vi "Lab_JouleScope.vi"() -> ()   [LabVIEW 2015]
uses:
  Ctrl/I_range.ctl
  Ctrl/R_W.ctl
  <vilib>/Analysis/3filter.llb/Filter Passband Type.ctl
  SubVIs/JSON_send/Send_JSN_Message_2 (SubVI).vi
  SubVIs/JSON_send/Send_JSN_Message_0 (SubVI).vi
  SubVIs/JSON_extract_data/JSON_extract_Data_2 (SubVI).vi
  SubVIs/JSON_extract_data/JSON_extract_Data_1 (SubVI).vi
  SubVIs/JSON_send/Send_JSN_Message_1 (SubVI).vi
  SubVIs/JSON_extract_data/JSON_extract_Data_7 (SubVI).vi
  SubVIs/JSON_extract_data/JSON_extract_Data_6 (SubVI).vi
  SubVIs/JSON_send/Send_JSN_Message_7 (SubVI).vi
  SubVIs/JSON_extract_data/JSON_extract_Data_4 (SubVI).vi
  <vilib>/Analysis/3filter.llb/Butterworth Filter (DBL).vi
  <vilib>/Analysis/NI_AALBase.lvlib
panel:
  out "Stop_Var":bool=TRUE
  in  "Tab Control":enum32{"Init", "Visu"}(tab)=enum."Visu"
  out "Device":string="Joulescope:001747"
  out "Parameters":string="{\"type\": \"parameters\", \"phase\": \"rsp\", \"id\": 3, \"status\": 200, \"status_msg\": \"Success\", \"device\": \"Joulescope:001747\", \"data\": {\"sensor_power\": {\"name\": \"sensor_power\", \"default\": \"on\", \"path\": \"setting\", \"options\": [[\"off\", 0, []], [\"on\", 1, []]], \"units\": null, \"brief\": \"Force the sensor power on or off.\", \"detail\": \"Altering this parameter during operation may cause errors.\", \"flags\": [\"developer\"]}, \"source\": {\"name\": \"source\", \"default\": \"off\", \"path\": \"setting\", \"options\": [[\"off\", 0, []], [\"raw\", 192, [\"on\"]], [\"pattern_usb\", 9, []], [\"pattern_control\", 10, []], [\"pattern_sensor\", 175, []]], \"units\": null, \"brief\": \"Select the streaming data source.\", \"detail\": null, \"flags\": [\"developer\"]}, \"i_range\": {\"name\": \"i_range\", \"default\": \"off\", \"path\": \"setting\", \"options\": [[\"auto\", 128, [\"on\"]], [\"10 A\", 1, [\"0\", 0]], [\"2 A\", 2, [\"1\", 1]], [\"180 mA\", 4, [\"2\", 2]], [\"18 mA\", 8, [\"3\", 3]], [\"1.8 mA\", 16, [\"4\", 4]], [\"180 \\u00b5A\", 32, [\"5\", 5]], [\"18 \\u00b5A\", 64, [\"6\", 6]], [\"off\", 0, []]], \"units\": null, \"brief\": \"Select the current measurement range (shunt resistor)\", \"detail\": null, \"flags\": []}, \"v_range\": {\"name\": \"v_range\", \"default\": \"15V\", \"path\": \"setting\", \"options\": [[\"15V\", 0, [\"low\", 0]], [\"5V\", 1, [\"high\", 1]]], \"units\": null, \"brief\": \"Select the voltage measurement range (gain)\", \"detail\": null, \"flags\": []}, \"ovr_to_lsb\": {\"name\": \"ovr_to_lsb\", \"default\": \"off\", \"path\": \"setting\", \"options\": [[\"off\", 0, []], [\"on\", 1, []]], \"units\": null, \"brief\": \"Map overflow flags to the LSBs\", \"detail\": null, \"flags\": [\"developer\"]}, \"trigger_source\": {\"name\": \"trigger_source\", \"default\": \"auto\", \"path\": \"extio\", \"options\": [[\"auto\", 0, []], [\"gpi0\", 2, []], [\"gpi1\", 3, []]], \"units\": null, \"brief\": \"Select the trigger source\", \"detail\": null, \"flags\": [\"hidden\"]}, \"io_voltage\": {\"name\": \"io_voltage\", \"default\": \"3.3V\", \"path\": \"extio\", \"options\": [[\"1.8V\", 1800, []], [\"2.1V\", 2100, []], [\"2.5V\", 2500, []], [\"2.7V\", 2700, []], [\"3.0V\", 3000, []], [\"3.3V\", 3300, []], [\"3.6V\", 3600, []], [\"5.0V\", 5000, []]], \"units\": null, \"brief\": \"The GPI/O high-level voltage.\", \"detail\": null, \"flags\": []}, \"gpo0\": {\"name\": \"gpo0\", \"default\": \"0\", \"path\": \"extio\", \"options\": [[\"0\", 0, [0]], [\"1\", 1, [1]]], \"units\": null, \"brief\": \"The GPO bit 0 output value.\", \"detail\": null, \"flags\": []}, \"gpo1\": {\"name\": \"gpo1\", \"default\": \"0\", \"path\": \"extio\", \"options\": [[\"0\", 0, [0]], [\"1\", 1, [1]]], \"units\": null, \"brief\": \"The GPO bit 1 output value.\", \"detail\": null, \"flags\": []}, \"current_lsb\": {\"name\": \"current_lsb\", \"default\": \"normal\", \"path\": \"extio\", \"options\": [[\"normal\", 0, []], [\"gpi0\", 2, []], [\"gpi1\", 3, []]], \"units\": null, \"brief\": \"The current signal least-significant bit mapping.\", \"detail\": null, \"flags\": []}, \"voltage_lsb\": {\"name\": \"voltage_lsb\", \"default\": \"normal\", \"path\": \"extio\", \"options\": [[\"normal\", 0, []], [\"gpi0\", 2, []], [\"gpi1\", 3, []]], \"units\": null, \"brief\": \"The voltage signal least-significant bit mapping.\", \"detail\": null, \"flags\": []}, \"control_test_mode\": {\"name\": \"control_test_mode\", \"default\": \"normal\", \"path\": \"setting\", \"options\": [[\"normal\", 3, []], [\"usb\", 129, []], [\"fpga\", 130, []], [\"both\", 131, []]], \"units\": null, \"brief\": \"Set the test mode\", \"detail\": null, \"flags\": [\"developer\"]}, \"transfer_length\": {\"name\": \"transfer_length\", \"default\": \"256\", \"path\": \"setting\", \"options\": [[\"1\", 1, []], [\"2\", 2, []], [\"4\", 4, []], [\"8\", 8, []], [\"16\", 16, []], [\"32\", 32, []], [\"64\", 64, []], [\"128\", 128, []], [\"256\", 256, []]], \"units\": \"packets\", \"brief\": \"Set the USB transfer length in packets\", \"detail\": null, \"flags\": [\"developer\", \"skip_update\"]}, \"transfer_outstanding\": {\"name\": \"transfer_outstanding\", \"default\": \"8\", \"path\": \"setting\", \"options\": [[\"1\", 1, []], [\"2\", 2, []], [\"4\", 4, []], [\"8\", 8, []]], \"units\": null, \"brief\": \"Set the maximum number of USB transfers issued simultaneously\", \"detail\": null, \"flags\": [\"developer\", \"skip_update\"]}, \"current_ranging\": {\"name\": \"current_ranging\", \"default\": null, \"path\": \"current_ranging\", \"options\": [], \"units\": null, \"brief\": null, \"detail\": null, \"flags\": [\"hidden\"]}, \"current_ranging_type\": {\"name\": \"current_ranging_type\", \"default\": \"interp\", \"path\": \"current_ranging\", \"options\": [[\"off\", \"off\", []], [\"mean\", \"mean\", []], [\"interp\", \"interp\", [\"interpolate\"]], [\"NaN\", \"nan\", [\"nan\"]]], \"units\": null, \"brief\": \"The filter type.\", \"detail\": null, \"flags\": []}, \"current_ranging_samples_pre\": {\"name\": \"current_ranging_samples_pre\", \"default\": \"1\", \"path\": \"current_ranging\", \"options\": [[\"0\", 0, [0]], [\"1\", 1, [1]], [\"2\", 2, [2]], [\"3\", 3, [3]], [\"4\", 4, [4]], [\"5\", 5, [5]], [\"6\", 6, [6]], [\"7\", 7, [7]], [\"8\", 8, [8]]], \"units\": null, \"brief\": \"The number of samples before the range switch to include.\", \"detail\": \"Only valid for type \\\"mean\\\" - ignored for \\\"off\\\", \\\"interp\\\", and \\\"NaN\\\".\", \"flags\": []}, \"current_ranging_samples_window\": {\"name\": \"current_ranging_samples_window\", \"default\": \"n\", \"path\": \"current_ranging\", \"options\": [[\"m\", \"m\", []], [\"n\", \"n\", []], [\"0\", 0, [0]], [\"1\", 1, [1]], [\"2\", 2, [2]], [\"3\", 3, [3]], [\"4\", 4, [4]], [\"5\", 5, [5]], [\"6\", 6, [6]], [\"7\", 7, [7]], [\"8\", 8, [8]], [\"9\", 9, [9]], [\"10\", 10, [10]], [\"11\", 11, [11]], [\"12\", 12, [12]]], \"units\": null, \"brief\": \"The number of samples to adjust.\", \"detail\": \"Use \\\"n\\\" for automatic duration based upon known response time. Use \\\"m\\\" for shorter automatic duration that may result in min/max distortion.\", \"flags\": []}, \"current_ranging_samples_post\": {\"name\": \"current_ranging_samples_post\", \"default\": \"1\", \"path\": \"current_ranging\", \"options\": [[\"0\", 0, [0]], [\"1\", 1, [1]], [\"2\", 2, [2]], [\"3\", 3, [3]], [\"4\", 4, [4]], [\"5\", 5, [5]], [\"6\", 6, [6]], [\"7\", 7, [7]], [\"8\", 8, [8]]], \"units\": null, \"brief\": \"The number of samples after the range switch to include.\", \"detail\": \"Only valid for type \\\"mean\\\" - ignored for \\\"off\\\", \\\"interp\\\", and \\\"NaN\\\".\", \"flags\": []}, \"buffer_duration\": {\"name\": \"buffer_duration\", \"default\": \"30 seconds\", \"path\": \"setting\", \"options\": [[\"15 seconds\", 15, [15]], [\"30 seconds\", 30, [30]], [\"1 minute\", 60, [60]], [\"2 minutes\", 120, [120]], [\"5 minutes\", 300, [300]], [\"10 minutes\", 600, [600]], [\"20 minutes\", 1200, [1200]], [\"1 hour\", 3600, [3600]], [\"2 hours\", 7200, [7200]], [\"5 hours\", 18000, [18000]], [\"10 hours\", 36000, [36000]], [\"1 day\", 86400, [86400]]], \"units\": \"seconds\", \"brief\": \"The amount of sample data to store in memory.\", \"detail\": \"Use care when setting this value. The software requires 1.5 GB of RAM for every 60 seconds at the full 2 MSPS rate.\", \"flags\": [\"skip_update\"]}, \"reduction_frequency\": {\"name\": \"reduction_frequency\", \"default\": \"2 Hz\", \"path\": \"setting\", \"options\": [[\"100 Hz\", 100, [100]], [\"50 Hz\", 50, [50]], [\"20 Hz\", 20, [20]], [\"10 Hz\", 10, [10]], [\"5 Hz\", 5, [5]], [\"2 Hz\", 2, [2]], [\"1 Hz\", 1, [1]]], \"units\": \"Hz\", \"brief\": \"The rate that the device produces statistics, including multimeter values.\", \"detail\": null, \"flags\": [\"skip_update\"]}, \"sampling_frequency\": {\"name\": \"sampling_frequency\", \"default\": \"2 MHz\", \"path\": \"setting\", \"options\": [[\"2 MHz\", 2000000, [2000000, \"auto\", null, \"default\"]], [\"1 MHz\", 1000000, [1000000]], [\"500 kHz\", 500000, [500000]], [\"200 kHz\", 200000, [200000]], [\"100 kHz\", 100000, [100000]], [\"50 kHz\", 50000, [50000]], [\"20 kHz\", 20000, [20000]], [\"10 kHz\", 10000, [10000]], [\"5 kHz\", 5000, [5000]], [\"2 kHz\", 2000, [2000]], [\"1 kHz\", 1000, [1000]], [\"500 Hz\", 500, [500]], [\"200 Hz\", 200, [200]], [\"100 Hz\", 100, [100]], [\"50 Hz\", 50, [50]], [\"20 Hz\", 20, [20]], [\"10 Hz\", 10, [10]]], \"units\": \"Hz\", \"brief\": \"The rate that the device produces samples.\", \"detail\": null, \"flags\": [\"skip_update\"]}, \"model\": {\"name\": \"model\", \"default\": null, \"path\": \"info\", \"options\": [], \"units\": null, \"brief\": null, \"detail\": null, \"flags\": [\"read_only\", \"hidden\"]}, \"device_serial_number\": {\"name\": \"device_serial_number\", \"default\": null, \"path\": \"info\", \"options\": [], \"units\": null, \"brief\": null, \"detail\": null, \"flags\": [\"read_only\", \"hidden\"]}, \"hardware_serial_number\": {\"name\": \"hardware_serial_number\", \"default\": null, \"path\": \"info\", \"options\": [], \"units\": null, \"brief\": null, \"detail\": null, \"flags\": [\"read_only\", \"hidden\"]}}}"
  out "Infos":T1={"protocol_version"=1, "server_version"="0.1.2", "joulescope_version"="0.9.7"}
  out "infos":string="{\"type\": \"info\", \"phase\": \"rsp\", \"id\": 4, \"status\": 200, \"status_msg\": \"Success\", \"device\": \"Joulescope:001747\", \"data\": {\"type\": \"info\", \"ver\": 1, \"ctl\": {\"mfg\": {\"country\": \"USA\", \"location\": \"MD_01\", \"lot\": \"202043_00\"}, \"hw\": {\"rev\": \"H\", \"sn_mcu\": \"510D00D070D4A1BA683523C52091005F\", \"sn_mfg\": \"001747\"}, \"fw\": {\"ver\": \"1.3.2\"}, \"fpga\": {\"ver\": \"0.2.0\", \"prod_id\": \"0x9314acf2\"}}, \"sensor\": {\"fw\": {\"ver\": \"1.3.2\"}, \"fpga\": {\"ver\": \"1.2.1\"}}}}"
  out "OK raw data":bool=TRUE
  in  "i_range request_1":cluster{"name":string, "value":T2}={"name"="i_range", "value"=enum."1.8 mA"}
  out "Current":sgl[](graph)
  out "Voltage":sgl[](graph)
  in  "fc":dbl=2000.0 format="%#_13g"
  in  "stop":bool
  out "i_range":string="1.8 mA"
  out "statistiques":string="{\"type\": \"statistics\", \"phase\": \"async\", \"device\": \"Joulescope:001747\", \"data\": {\"time\": {\"range\": {\"value\": [29.0, 29.5], \"units\": \"s\"}, \"delta\": {\"value\": 0.5, \"units\": \"s\"}, \"samples\": {\"value\": 1000000, \"units\": \"samples\"}, \"sample_range\": {\"value\": [58000000, 59000000], \"units\": \"input_samples\"}}, \"signals\": {\"current\": {\"\\u00b5\": {\"value\": 2.5195384097245923e-06, \"units\": \"A\"}, \"\\u03c32\": {\"value\": 1.3499273425982267e-11, \"units\": \"A\"}, \"min\": {\"value\": -1.4949010619602632e-05, \"units\": \"A\"}, \"max\": {\"value\": 3.776274752453901e-05, \"units\": \"A\"}, \"p2p\": {\"value\": 5.271175814414164e-05, \"units\": \"A\"}, \"\\u222b\": {\"value\": 1.2597692048622961e-06, \"units\": \"C\"}}, \"voltage\": {\"\\u00b5\": {\"value\": 2.988984020348548, \"units\": \"V\"}, \"\\u03c32\": {\"value\": 1.098181211591936e-06, \"units\": \"V\"}, \"min\": {\"value\": 2.984358787536621, \"units\": \"V\"}, \"max\": {\"value\": 2.993438720703125, \"units\": \"V\"}, \"p2p\": {\"value\": 0.009079933166503906, \"units\": \"V\"}}, \"power\": {\"\\u00b5\": {\"value\": 7.5309005292030786e-06, \"units\": \"W\"}, \"\\u03c32\": {\"value\": 1.206049847016679e-10, \"units\": \"W\"}, \"min\": {\"value\": -4.4664109736913815e-05, \"units\": \"W\"}, \"max\": {\"value\": 0.00011286902736173943, \"units\": \"W\"}, \"p2p\": {\"value\": 0.00015753313709865324, \"units\": \"W\"}, \"\\u222b\": {\"value\": 3.7654502646015393e-06, \"units\": \"J\"}}, \"current_range\": {\"\\u00b5\": {\"value\": 4.0, \"units\": \"\"}, \"\\u03c32\": {\"value\": 0.0, \"units\": \"\"}, \"min\": {\"value\": 4.0, \"units\": \"\"}, \"max\": {\"value\": 4.0, \"units\": \"\"}, \"p2p\": {\"value\": 0.0, \"units\": \"\"}}, \"current_lsb\": {\"\\u00b5\": {\"value\": 0.5333319999999999, \"units\": \"\"}, \"\\u03c32\": {\"value\": 0.24888922666522673, \"units\": \"\"}, \"min\": {\"value\": 0.0, \"units\": \"\"}, \"max\": {\"value\": 1.0, \"units\": \"\"}, \"p2p\": {\"value\": 1.0, \"units\": \"\"}}, \"voltage_lsb\": {\"\\u00b5\": {\"value\": 0.5333329999999997, \"units\": \"\"}, \"\\u03c32\": {\"value\": 0.24888916000015993, \"units\": \"\"}, \"min\": {\"value\": 0.0, \"units\": \"\"}, \"max\": {\"value\": 1.0, \"units\": \"\"}, \"p2p\": {\"value\": 1.0, \"units\": \"\"}}}, \"source\": \"stream_buffer\", \"accumulators\": {\"charge\": {\"value\": 7.7435459e-05, \"units\": \"C\"}, \"energy\": {\"value\": 0.00023147490999999998, \"units\": \"J\"}}}, \"status\": 200, \"status_msg\": \"Success\"}"
  # "Lab_JouleScope"
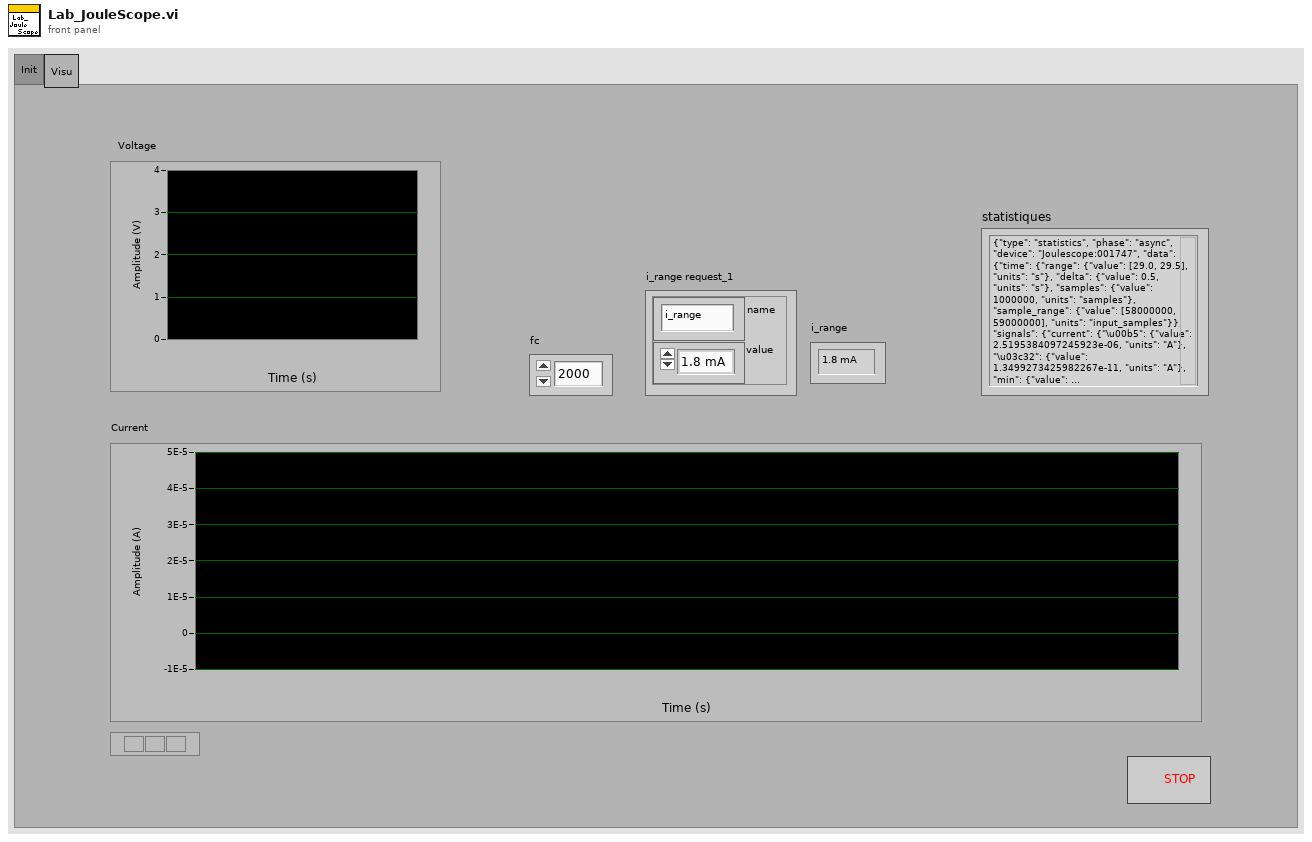
[diagram p1: front panel]
types:
  T1 = cluster{"protocol_version":i32, "server_version":string, "joulescope_version":string}
  T2 = typedef "I_range.ctl" = enum16{"off", "18 µA", "180 µA", "1.8 mA", "18 mA", "180 mA", "2 A", "10 A", "auto"}
  T3 = typedef "R_W.ctl" = enum16{"Write", "Read", "RAZ"}
  T4 = typedef "NI_AALBase.lvlib/Filter Passband Type.ctl" = enum32{"Lowpass", "Highpass", "Bandpass", "Bandstop"}
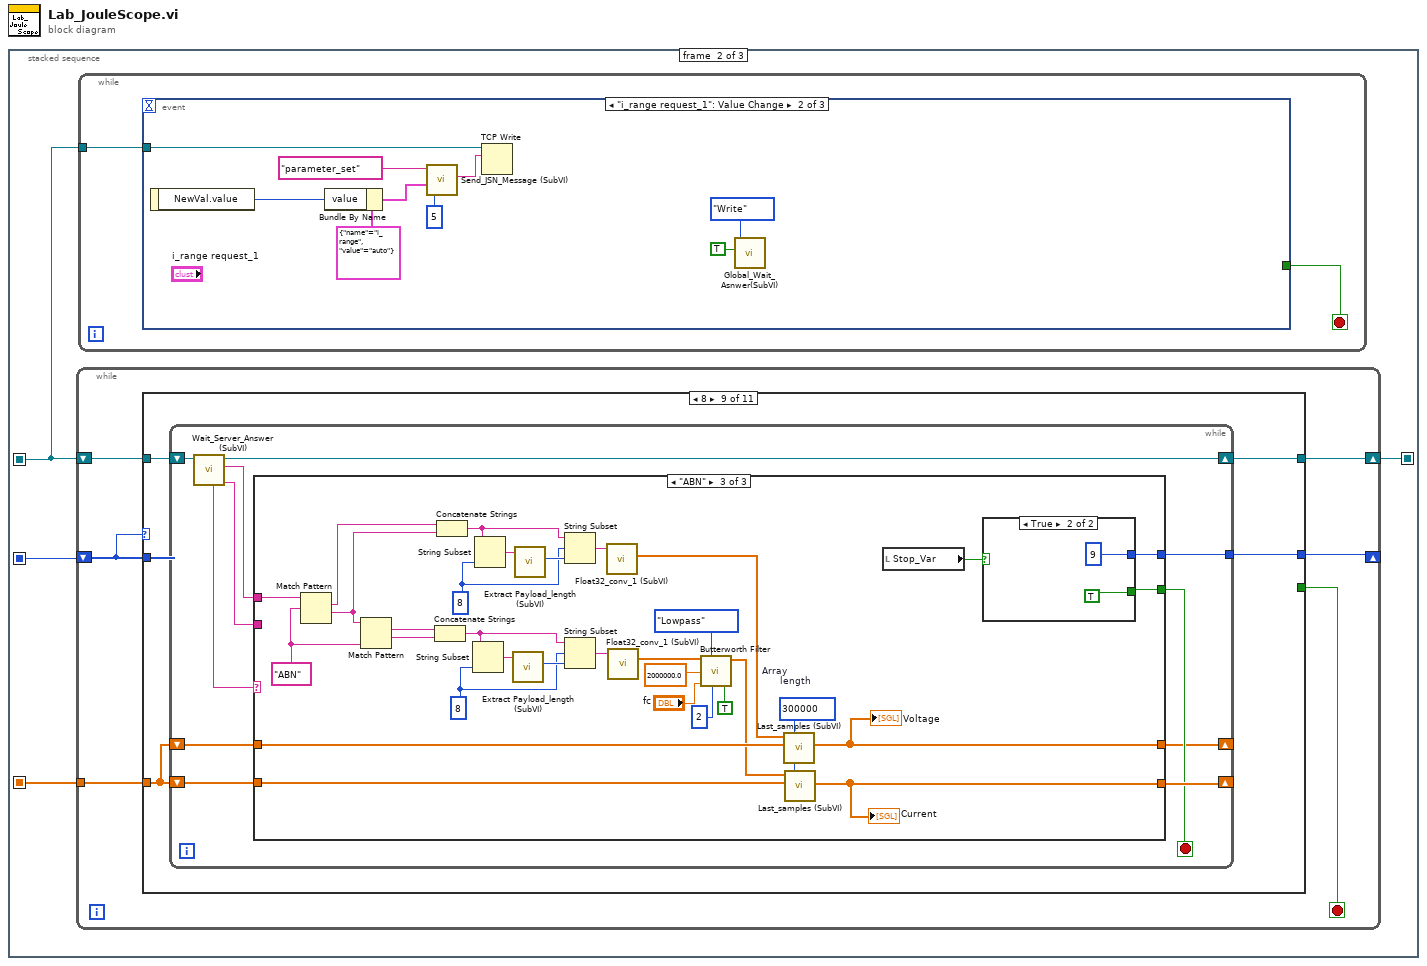
[diagram p0: block diagram]
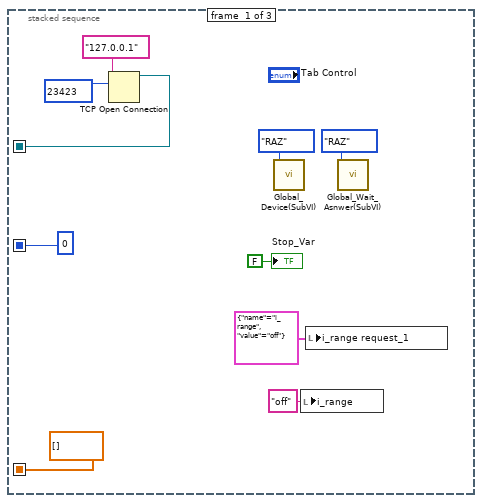
[diagram p2: hidden frame]
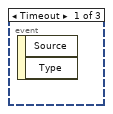
[diagram p3: hidden frame]
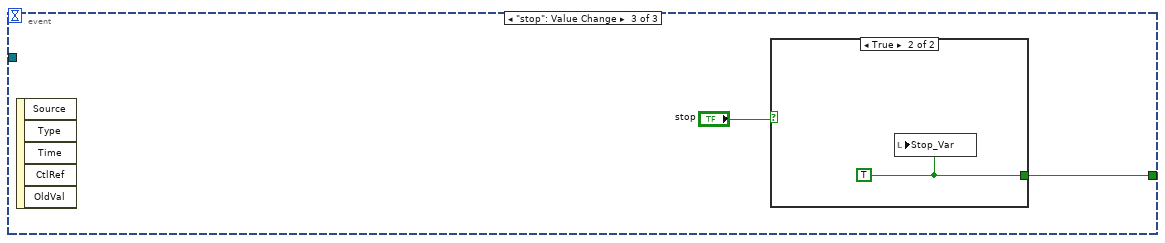
[diagram p4: hidden frame]
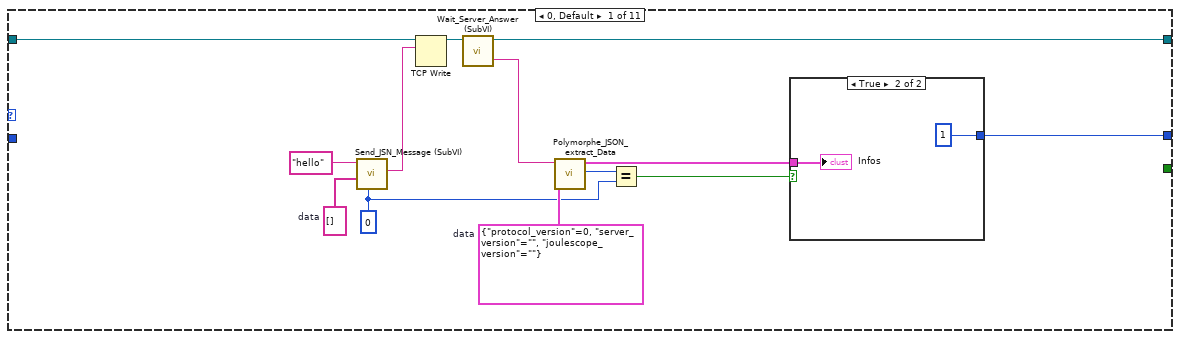
[diagram p6: hidden frame]
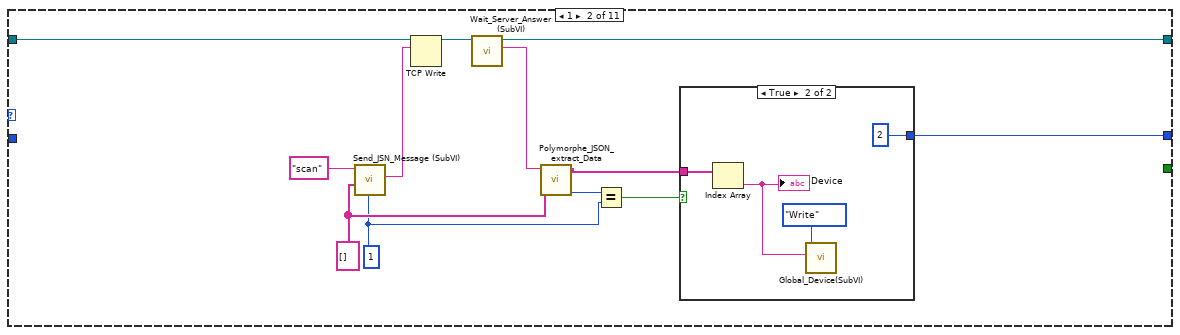
[diagram p8: hidden frame]
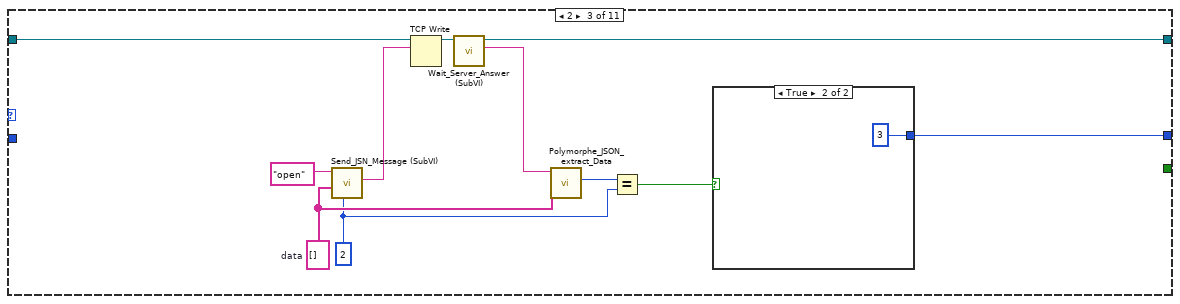
[diagram p10: hidden frame]
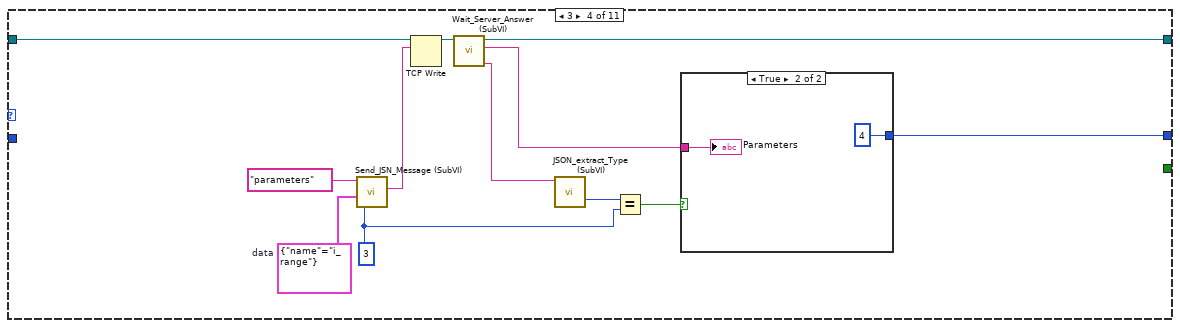
[diagram p12: hidden frame]
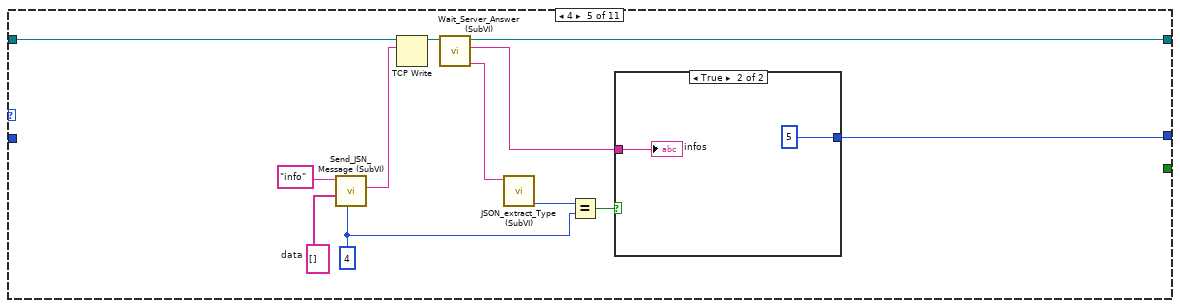
[diagram p14: hidden frame]
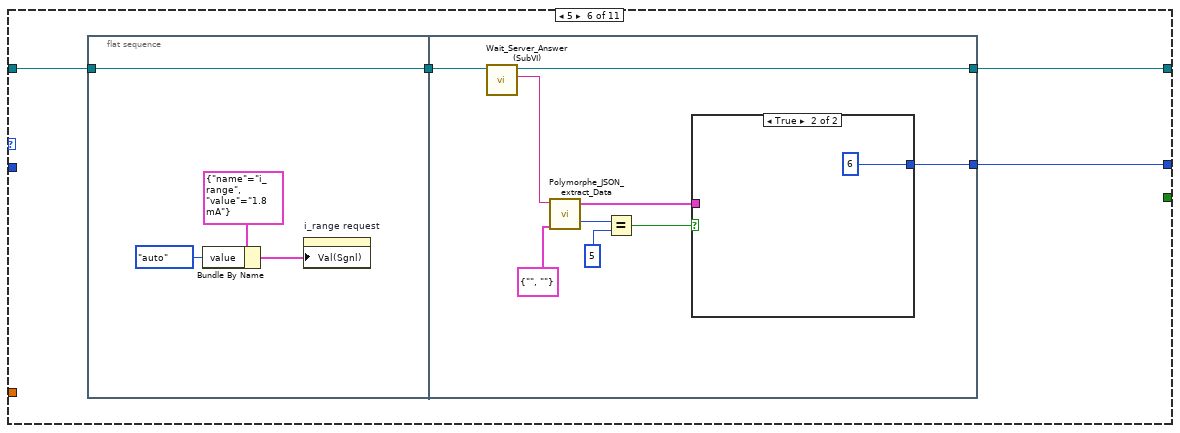
[diagram p16: hidden frame]
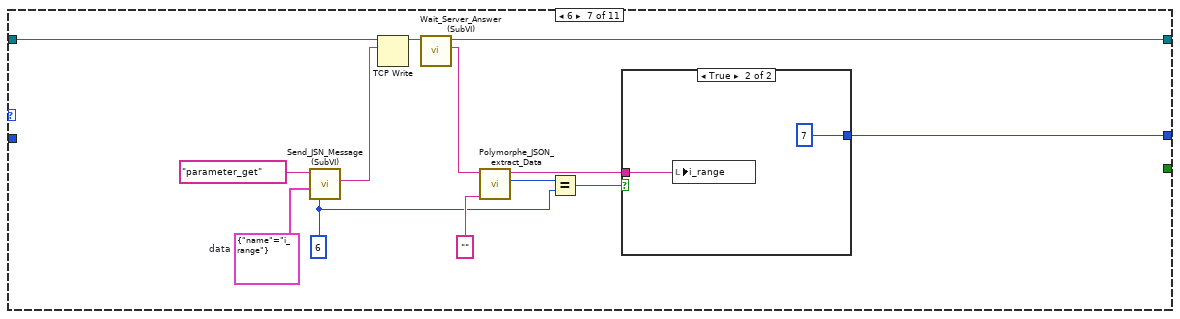
[diagram p18: hidden frame]
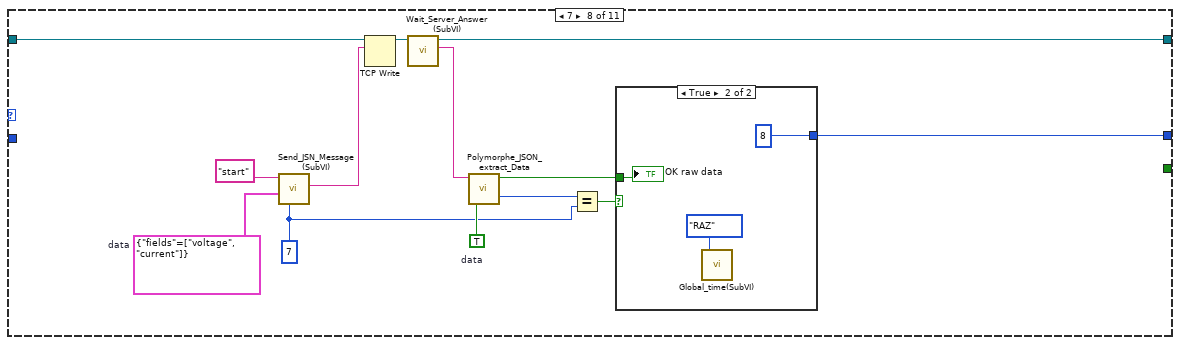
[diagram p20: hidden frame]
diagram:
  n1 = stacked-sequence {
    seq-local: [w8 _ _] -> [_ w11 _]
    seq-local: [0 _ _] -> [_ w14 _]
    seq-local: [_ w13 _] -> [_ _ w257]
    seq-local: [sgl[] [] _ _] -> [_ w12 _]
    frame #0 {
      n2 = TCP Open Connection(address="127.0.0.1", remote port or service name=u16 23423) -> (connection ID=w8:refnum<k5>)  [unwired: 3 in, 1 out]
      n3 = call "Global_Device(SubVI).vi"("R/W"=R_W."RAZ") -> ()  [unwired: 10 in, 1 out]
      n4 = local write "i_range"("off" ("i_range")) -> ()
      n5 = local write "i_range request_1"(cluster{"name":string, "value":T2} {"name"="i_range", "value"=enum."off"} ("i_range request_1")) -> ()
      n6 = call "Global_Wait_Asnwer(SubVI).vi"("R/W"=R_W."RAZ") -> ()  [unwired: 10 in, 1 out]
      "Stop_Var" <- FALSE ("Stop_Var")
    }
    frame #1 {
      n7 = while {
        shift-right: [w31] -> w13
        shift-left: w11 -> [w34]
        shift-right: [w32] -> _
        shift-left: w14 -> [w33]
        tunnel: w12 -> [w29]
        stop <- w30 stop-if-true
        n8 = case shown="8" w33 {
          tunnel: w34 -> [w47 w61 w76 w89 w103 w109 w136 w151 w157 w234 w249]
          tunnel: [w45 w59 w75 w88 w102 w108 w135 w150 w158 w233 w250] -> w31
          tunnel: w33 -> [_ _ _ _ _ _ _ _ _ _ _]
          tunnel: [w44 w58 w74 w87 w96 w107 w132 w149 w156 w231 _] -> w32
          tunnel: [_ _ _ _ _ _ _ _ _ _ w248] -> w30
          tunnel: w29 -> [_ _ _ _ _ _ _ _ w155 _ _]
          frame 0, Default {
            w35 = string[] []  # data
            w41 = T1 {"protocol_version"=0, "server_version"="", "joulescope_version"=""}  # data
            w36 = 0 ("device")
            n9 = call-poly "Send_JSN_Message (SubVI).vi"("id"=w36, "data"=w35, "type"="hello") -> ("JSON message"=w38:string)  [unwired: 7 in, 1 out]
            n10 = TCP Write(connection ID=w47, data in=w38) -> (connection ID out=w46:refnum<k5>)  [unwired: 2 in, 2 out]
            n11 = call "Wait_Server_Answer (SubVI).vi"("TCP Network Connection in"=w46) -> ("data out"=w42:string, "TCP Network Connection out"=w45:refnum<k5>)  [unwired: 7 in, 2 out]
            n12 = call-poly "Polymorphe_JSON_extract_Data.vi"("data"=w41, "cluster in"=w42) -> ("id"=w40:u8, "data"=w39:T1)  [unwired: 8 in]
            n13 = Equal?(x=w40, y=w36) -> (x = y?=w43:bool)
            n14 = case shown="True" w43 {
              tunnel: [_ 1] -> w44
              tunnel: w39 -> [_ w48]
              frame False {
              }
              frame True {
                "Infos" <- w48
              }
            }
          }
          frame 1 {
            w51 = string[] [] ("data")
            w50 = 1 ("device")
            n15 = call-poly "Send_JSN_Message (SubVI).vi"("id"=w50, "data"=w51, "type"="scan") -> ("JSON message"=w53:string)  [unwired: 7 in, 1 out]
            n16 = TCP Write(connection ID=w61, data in=w53) -> (connection ID out=w60:refnum<k5>)  [unwired: 2 in, 2 out]
            n17 = call "Wait_Server_Answer (SubVI).vi"("TCP Network Connection in"=w60) -> ("data out"=w56:string, "TCP Network Connection out"=w59:refnum<k5>)  [unwired: 7 in, 2 out]
            n18 = call-poly "Polymorphe_JSON_extract_Data.vi"("data type"=w51, "Response in"=w56) -> ("id"=w54:u8, "Response out"=w55:string[])  [unwired: 8 in]
            n19 = Equal?(x=w54, y=w50) -> (x = y?=w57:bool)
            n20 = case shown="True" w57 {
              tunnel: [_ 2] -> w58
              tunnel: w55 -> [_ w64]
              frame False {
              }
              frame True {
                n21 = Index Array(array=w64) -> (element=w62:string)  [unwired: 1 in]
                "Device" <- w62
                n22 = call "Global_Device(SubVI).vi"("Device in"=w62, "R/W"=R_W."Write") -> ()  [unwired: 9 in, 1 out]
              }
            }
          }
          frame 2 {
            w67 = string[] []  # data
            w66 = 2 ("device")
            n23 = call-poly "Send_JSN_Message (SubVI).vi"("id"=w66, "data"=w67, "type"="open") -> ("JSON message"=w69:string)  [unwired: 7 in, 1 out]
            n24 = TCP Write(connection ID=w76, data in=w69) -> (connection ID out=w73:refnum<k5>)  [unwired: 2 in, 2 out]
            n25 = call "Wait_Server_Answer (SubVI).vi"("TCP Network Connection in"=w73) -> ("data out"=w72:string, "TCP Network Connection out"=w75:refnum<k5>)  [unwired: 7 in, 2 out]
            n26 = call-poly "Polymorphe_JSON_extract_Data.vi"("data type"=w67, "Response in"=w72) -> ("id"=w71:u8)  [unwired: 8 in, 1 out]
            n27 = Equal?(x=w71, y=w66) -> (x = y?=w70:bool)
            n28 = case shown="True" w70 {
              tunnel: [_ 3] -> w74
              frame False {
              }
              frame True {
              }
            }
          }
          frame 3 {
            w80 = cluster{"name":string} {"name"="i_range"}  # data
            w78 = 3 ("device")
            n29 = call-poly "Send_JSN_Message (SubVI).vi"("id"=w78, "data"=w80, "type"="parameters") -> ("JSON message"=w81:string)  [unwired: 8 in]
            n30 = TCP Write(connection ID=w89, data in=w81) -> (connection ID out=w86:refnum<k5>)  [unwired: 2 in, 2 out]
            n31 = call "Wait_Server_Answer (SubVI).vi"("TCP Network Connection in"=w86) -> ("total_message"=w85:string, "data out"=w82:string, "TCP Network Connection out"=w88:refnum<k5>)  [unwired: 7 in, 1 out]
            n32 = call "JSON_extract_Type (SubVI).vi"("data in"=w85) -> ("id"=w84:i32)  [unwired: 9 in, 1 out]
            n33 = Equal?(x=w84, y=w78) -> (x = y?=w83:bool)
            n34 = case shown="True" w83 {
              tunnel: [_ 4] -> w87
              tunnel: w82 -> [_ w90]
              frame False {
              }
              frame True {
                "Parameters" <- w90
              }
            }
          }
          frame 4 {
            w94 = string[] []  # data
            w92 = 4 ("device")
            n35 = call-poly "Send_JSN_Message (SubVI).vi"("id"=w92, "data"=w94, "type"="info") -> ("JSON message"=w95:string)  [unwired: 7 in, 1 out]
            n36 = TCP Write(connection ID=w103, data in=w95) -> (connection ID out=w101:refnum<k5>)  [unwired: 2 in, 2 out]
            n37 = call "Wait_Server_Answer (SubVI).vi"("TCP Network Connection in"=w101) -> ("total_message"=w97:string, "data out"=w98:string, "TCP Network Connection out"=w102:refnum<k5>)  [unwired: 7 in, 1 out]
            n38 = call "JSON_extract_Type (SubVI).vi"("data in"=w97) -> ("id"=w100:i32)  [unwired: 9 in, 1 out]
            n39 = Equal?(x=w100, y=w92) -> (x = y?=w99:bool)
            n40 = case shown="True" w99 {
              tunnel: [_ 5] -> w96
              tunnel: w98 -> [_ w104]
              frame False {
              }
              frame True {
                "infos" <- w104
              }
            }
          }
          frame 5 {
            n41 = flat-sequence {
              tunnel: w109 -> [w113]
              tunnel: [w113] -> w106
              tunnel: [w121] -> w108
              tunnel: [w115] -> w107
              tunnel: w106 -> [w122]
              frame #0 {
                n42 = Bundle By Name(cluster=cluster{"name":string, "value":T2} {"name"="i_range", "value"=enum."1.8 mA"} ("i_range request"), "value"=I_range."auto") -> (w112:cluster{"name":string, "value":T2})
                n43 = property on="i_range request" class="Clust (strict)"("Val(Sgnl)"=w112) -> ()  [unwired: 2 in, 2 out]
              }
              frame #1 {
                n44 = call "Wait_Server_Answer (SubVI).vi"("TCP Network Connection in"=w122) -> ("data out"=w117:string, "TCP Network Connection out"=w121:refnum<k5>)  [unwired: 7 in, 2 out]
                n45 = call-poly "Polymorphe_JSON_extract_Data.vi"("Data type"=cluster{"name":string, "value":string} {"name"="", "value"=""} ("data"), "Response in"=w117) -> ("id"=w119:u8, "Response out"=w118:cluster{"name":string, "value":string})  [unwired: 8 in]
                n46 = Equal?(x=w119, y=5 ("device")) -> (x = y?=w120:bool)
                n47 = case shown="True" w120 {
                  tunnel: [_ 6] -> w115
                  tunnel: w118 -> [_ _]
                  frame False {
                  }
                  frame True {
                  }
                }
              }
            }
          }
          frame 6 {
            w125 = cluster{"name":string} {"name"="i_range"}  # data
            w124 = 6 ("device")
            n48 = call-poly "Send_JSN_Message (SubVI).vi"("id"=w124, "data"=w125, "type"="parameter_get") -> ("JSON message"=w127:string)  [unwired: 8 in]
            n49 = TCP Write(connection ID=w136, data in=w127) -> (connection ID out=w134:refnum<k5>)  [unwired: 2 in, 2 out]
            n50 = call "Wait_Server_Answer (SubVI).vi"("TCP Network Connection in"=w134) -> ("data out"=w128:string, "TCP Network Connection out"=w135:refnum<k5>)  [unwired: 7 in, 2 out]
            n51 = call-poly "Polymorphe_JSON_extract_Data.vi"("data"="", "data in"=w128) -> ("id"=w131:u8, "data"=w130:string)  [unwired: 8 in]
            n52 = Equal?(x=w131, y=w124) -> (x = y?=w133:bool)
            n53 = case shown="True" w133 {
              tunnel: [_ 7] -> w132
              tunnel: w130 -> [_ w137]
              frame False {
              }
              frame True {
                n54 = local write "i_range"(w137) -> ()
              }
            }
          }
          frame 7 {
            w144 = TRUE  # data
            w146 = cluster{"fields":string[]} {"fields"=["voltage", "current"]}  # data
            w141 = 7 ("device")
            n55 = call-poly "Send_JSN_Message (SubVI).vi"("id"=w141, "data"=w146, "type"="start") -> ("JSON message"=w139:string)  [unwired: 8 in]
            n56 = TCP Write(connection ID=w151, data in=w139) -> (connection ID out=w148:refnum<k5>)  [unwired: 2 in, 2 out]
            n57 = call "Wait_Server_Answer (SubVI).vi"("TCP Network Connection in"=w148) -> ("data out"=w145:string, "TCP Network Connection out"=w150:refnum<k5>)  [unwired: 7 in, 2 out]
            n58 = call-poly "Polymorphe_JSON_extract_Data.vi"("data"=w144, "data in"=w145) -> ("id"=w142:u8, "data"=w143:bool)  [unwired: 8 in]
            n59 = Equal?(x=w142, y=w141) -> (x = y?=w147:bool)
            n60 = case shown="True" w147 {
              tunnel: [_ 8] -> w149
              tunnel: w143 -> [_ w153]
              frame False {
              }
              frame True {
                n61 = call "Global_time(SubVI).vi"("R/W"=enum16{"Write", "Read", "RAZ"}."RAZ") -> ()  [unwired: 10 in, 1 out]
                "OK raw data" <- w153
              }
            }
          }
          frame 8 {
            n62 = while {
              shift-right: [w165] -> w158
              shift-left: w157 -> [w169]
              tunnel: [w168] -> w156
              shift-right: [w166] -> _
              shift-left: w155 -> [w167]
              shift-right: [w159] -> _
              shift-left: w155 -> [w160]
              stop <- w163 stop-if-true
              n63 = call "Wait_Server_Answer (SubVI).vi"("TCP Network Connection in"=w169) -> ("total_message"=w161:string, "data out"=w164:string, "TCP Network Connection out"=w165:refnum<k5>, "Tag"=w162:string)  [unwired: 7 in]
              n64 = case shown="\"ABN\"" w162 {
                tunnel: [8 8 w220] -> w168
                tunnel: w167 -> [w176 w187 w219]
                tunnel: [w176 w187 w218] -> w166
                tunnel: w164 -> [w173 _ w212]
                tunnel: [_ _ w213] -> w163
                tunnel: w161 -> [w174 _ _]
                tunnel: w160 -> [w170 w186 w196]
                tunnel: [w170 w186 w195] -> w159
                frame "AJS" {
                  n65 = call "JSON_extract_Type (SubVI).vi"("data in"=w174) -> ("id"=w171:i32, "Type"=w172:string)  [unwired: 9 in]
                  n66 = case shown="Default" w172 {
                    tunnel: w171 -> [w180 _ _]
                    tunnel: w173 -> [w179 w185 _]
                    frame "parameter_set" {
                      n67 = Equal?(x=w180, y=5) -> (x = y?=w178:bool)
                      n68 = case shown="True" w178 {
                        tunnel: w179 -> [_ w184]
                        frame False {
                        }
                        frame True {
                          n69 = call-poly "Polymorphe_JSON_extract_Data.vi"("Data type"=cluster{"name":string, "value":string} {"name"="", "value"=""} ("data"), "Response in"=w184) -> ("Response out"=w182:cluster{"name":string, "value":string})  [unwired: 8 in, 1 out]
                          n70 = Unbundle By Name(w182) -> ("value"=→"i_range":string)
                        }
                      }
                    }
                    frame "statistics" {
                      "statistiques" <- w185
                    }
                    frame Default {
                    }
                  }
                }
                frame Default {
                }
                frame "ABN" {
                  w194 = 300000  # Array       length
                  w202 = 8 ("length (rest)")
                  w206 = 8 ("length (rest)")
                  w198 = "ABN" ("regular expression")
                  n71 = Match Pattern(string=w212, regular expression=w198) -> (match substring=w209:string, after substring=w207:string)  [unwired: 1 in, 2 out]
                  n72 = Match Pattern(string=w207, regular expression=w198) -> (match substring=w201:string, after substring=w200:string)  [unwired: 1 in, 2 out]
                  n73 = Concatenate Strings(w201, w200) -> (w203:string)
                  n74 = Concatenate Strings(w209, w207) -> (w208:string)
                  n75 = String Subset(string=w203, length (rest)=w202) -> (substring=w205:string)  [unwired: 1 in]
                  n76 = String Subset(string=w208, length (rest)=w206) -> (substring=w211:string)  [unwired: 1 in]
                  n77 = call "Extract Payload_length (SubVI).vi"("data in"=w205) -> ("Payload_length"=w204:u32)  [unwired: 8 in, 2 out]
                  n78 = call "Extract Payload_length (SubVI).vi"("data in"=w211) -> ("Payload_length"=w210:u32)  [unwired: 8 in, 2 out]
                  n79 = String Subset(string=w208, offset (0)=w206, length (rest)=w210) -> (substring=w217:string)
                  n80 = String Subset(string=w203, offset (0)=w202, length (rest)=w204) -> (substring=w199:string)
                  n81 = call "Float32_conv_1 (SubVI).vi"("data in"=w217) -> ("data out"=w197:sgl[])  [unwired: 10 in]
                  n82 = call "Float32_conv_1 (SubVI).vi"("data in"=w199) -> ("data out"=w191:sgl[])  [unwired: 10 in]
                  n83 = call-poly <vilib>:"Butterworth Filter.vi"("init/cont (init:F)"=TRUE, "order"=2, "filter type"=Filter_Passband_Type."Lowpass", "low cutoff freq: fl"="fc", "sampling freq: fs"=2000000.0, "X"=w191) -> ("Filtered X"=w190:dbl[])  [unwired: 2 in, 1 out]
                  n84 = call "Last_samples (SubVI).vi"("Array length"=w194, "Array in"=w196, "Samples in"=w197) -> ("Array out"=w195:sgl[])  [unwired: 8 in]
                  "Voltage" <- w195
                  n85 = call "Last_samples (SubVI).vi"("Array length"=w194, "Array in"=w219, "Samples in"=w190) -> ("Array out"=w218:sgl[])  [unwired: 8 in]
                  "Current" <- w218
                  n86 = local read "Stop_Var"() -> (w189:bool)
                  n87 = case shown="True" w189 {
                    tunnel: [_ 9] -> w220
                    tunnel: [_ TRUE] -> w213
                    frame False {
                    }
                    frame True {
                    }
                  }
                }
              }
            }
          }
          frame 9 {
            w224 = TRUE  # data
            w229 = string[] []  # data
            w227 = 10 ("device")
            w228 = "stop" ("type")
            n88 = call-poly "Send_JSN_Message (SubVI).vi"("id"=w227, "data"=w229, "type"=w228) -> ("JSON message"=w230:string)  [unwired: 7 in, 1 out]
            n89 = TCP Write(connection ID=w234, data in=w230) -> (connection ID out=w226:refnum<k5>)  [unwired: 2 in, 2 out]
            n90 = while {
              tunnel: w228 -> [w236]
              tunnel: [w238] -> w232
              shift-right: [w242] -> w233
              shift-left: w226 -> [w241]
              stop <- w240 stop-if-true
              n91 = call "Wait_Server_Answer (SubVI).vi"("TCP Network Connection in"=w241) -> ("total_message"=w239:string, "data out"=w238:string, "TCP Network Connection out"=w242:refnum<k5>)  [unwired: 7 in, 1 out]
              n92 = call "JSON_extract_Type (SubVI).vi"("data in"=w239) -> ("Type"=w237:string)  [unwired: 9 in, 1 out]
              n93 = Equal?(x=w237, y=w236) -> (x = y?=w240:bool)
            }
            n94 = call-poly "Polymorphe_JSON_extract_Data.vi"("data"=w224, "data in"=w232) -> ("id"=w225:u8)  [unwired: 8 in, 1 out]
            n95 = Equal?(x=w225, y=w227) -> (x = y?=w223:bool)
            n96 = case shown="True" w223 {
              tunnel: [_ 10] -> w231
              frame False {
              }
              frame True {
              }
            }
          }
          frame 10 {
            w244 = string[] []  # data
            w246 = "close" ("type")
            n97 = call-poly "Send_JSN_Message (SubVI).vi"("id"=11 ("device"), "data"=w244, "type"=w246) -> ("JSON message"=w243:string)  [unwired: 7 in, 1 out]
            n98 = TCP Write(connection ID=w249, data in=w243) -> (connection ID out=w247:refnum<k5>)  [unwired: 2 in, 2 out]
            n99 = while {
              tunnel: w246 -> [w252]
              tunnel: [w254] -> w248
              shift-right: [w253] -> w250
              shift-left: w247 -> [w256]
              stop <- w254 stop-if-true
              n100 = call "Wait_Server_Answer (SubVI).vi"("TCP Network Connection in"=w256) -> ("total_message"=w255:string, "TCP Network Connection out"=w253:refnum<k5>)  [unwired: 7 in, 2 out]
              n101 = call "JSON_extract_Type (SubVI).vi"("data in"=w255) -> ("Type"=w251:string)  [unwired: 9 in, 1 out]
              n102 = Equal?(x=w251, y=w252) -> (x = y?=w254:bool)
            }
          }
        }
      }
      n103 = while {
        tunnel: w11 -> [w16]
        stop <- w15 stop-if-true
        n104 = event shown="[1] \"i_range request_1\": Value Change" {
          selector: _ -> [_ _ _]
          dyn-events: _ -> [_ _ _]
          timeout: _ -> [_ _ _]
          tunnel: w16 -> [_ w25 _]
          tunnel: [_ _ w27] -> w15
          event Timeout {
            n105 = event-data() -> ()  [unwired: 1 in, 2 out]
          }
          event "i_range request_1": Value Change {
            n106 = event-data() -> ("NewVal.value"=w18:T2)  [unwired: 1 in]
            n107 = Bundle By Name(cluster=cluster{"name":string, "value":T2} {"name"="i_range", "value"=enum."auto"} ("i_range request"), "value"=w18) -> (w17:cluster{"name":string, "value":T2})
            n108 = call-poly "Send_JSN_Message (SubVI).vi"("id"=5 ("device"), "data"=w17, "type"="parameter_set") -> ("JSON message"=w22:string)  [unwired: 8 in]
            n109 = TCP Write(connection ID=w25, data in=w22) -> ()  [unwired: 2 in, 3 out]
            n110 = call "Global_Wait_Asnwer(SubVI).vi"("Wait_answer"=TRUE, "R/W"=R_W."Write") -> ()  [unwired: 9 in, 1 out]
          }
          event "stop": Value Change {
            n111 = event-data() -> ()  [unwired: 1 in, 5 out]
            n112 = case shown="True" "stop" {
              tunnel: [_ w28] -> w27
              frame False {
              }
              frame True {
                w28 = TRUE
                n113 = local write "Stop_Var"(w28) -> ()
              }
            }
          }
        }
      }
    }
    frame #2 {
      n114 = TCP Close Connection(connection ID=w257) -> ()  [unwired: 2 in, 2 out]
    }
  }
